vi "Tree_HierarchicalPath_Tests.vi"(11 "error in":errorcluster) -> (15 "error out":errorcluster)   [LabVIEW 2016, in "DronaTest.lvlib"]
uses:
  DronaTest.lvlib
  APIs/Stimulus/ControlValue/SetValueAuto.vi
  APIs/Stimulus/ControlValue/Controls/Tree/SetValueByHierarchicalPath.vi
  APIs/Assert/AssertControlValue/Equal.vi
  APIs/Get/GetControlRef/GetControlRefByPath.vi
  <vilib>/addons/_JKI Toolkits/Caraya/classes/Test/Test.lvclass
  Drona.lvlib
  <vilib>/SLL Toolkit/SLL Debug/SLL Debug.lvlib
  APIs/Assert/AssertControlValue/AssertControlValue.lvlib
  APIs/Stimulus/ControlValue/ControlValue.lvlib
  <vilib>/addons/_JKI Toolkits/Caraya/classes/Assert/Assert.lvclass
  APIs/Stimulus/ControlValue/Controls/Tree/StimulusTree.lvlib
  APIs/Get/GetControlRef/GetControlRef.lvlib
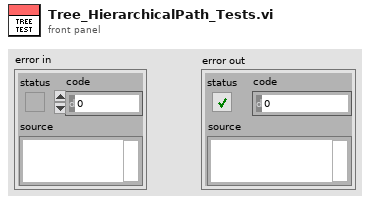
[diagram p1: front panel]
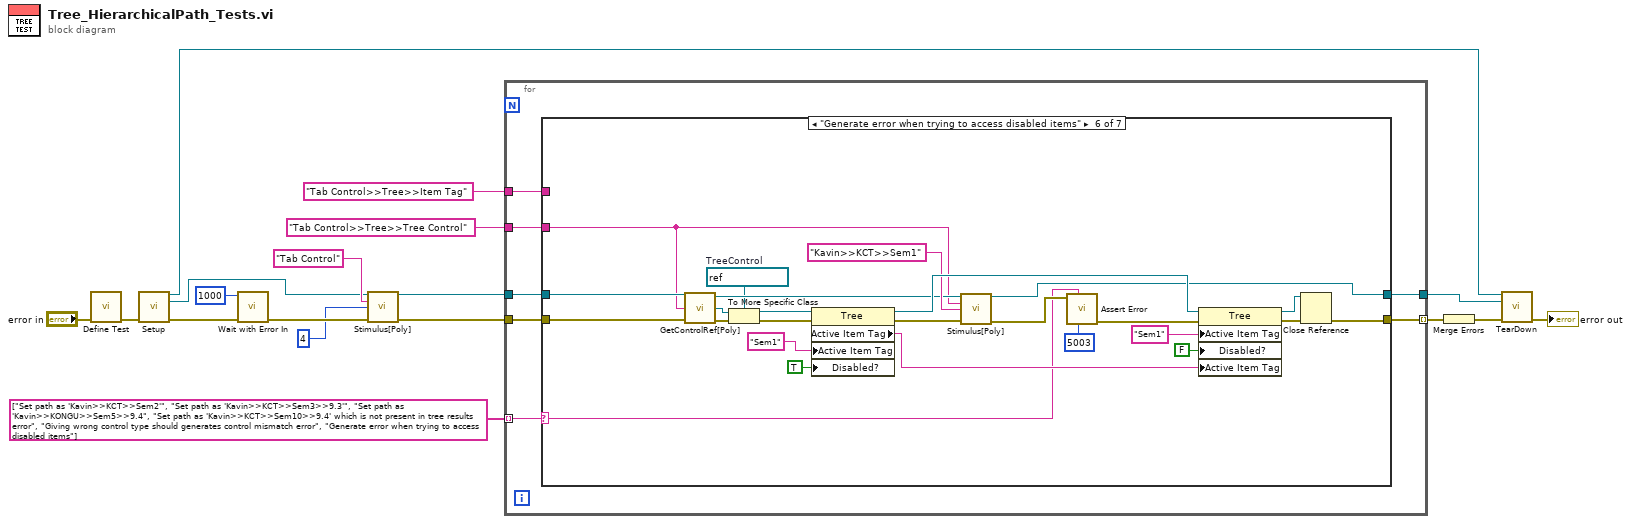
[diagram p0: block diagram]
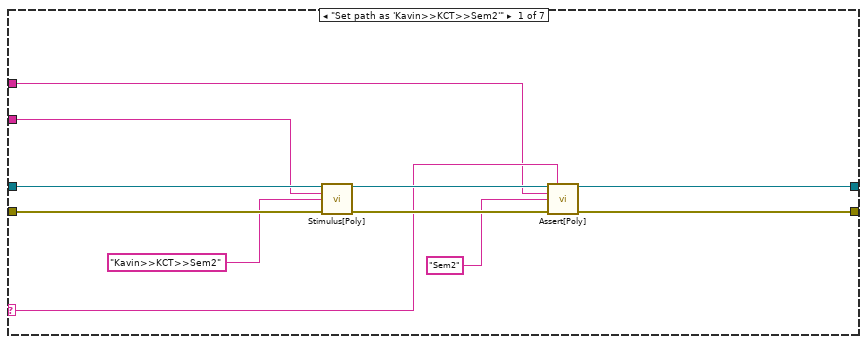
[diagram p2: hidden frame]
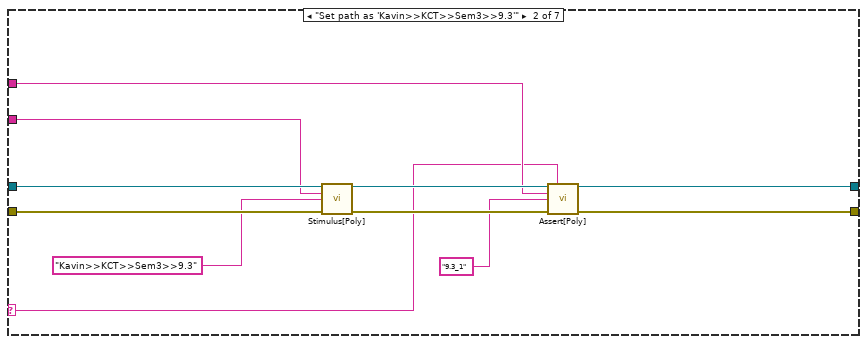
[diagram p3: hidden frame]
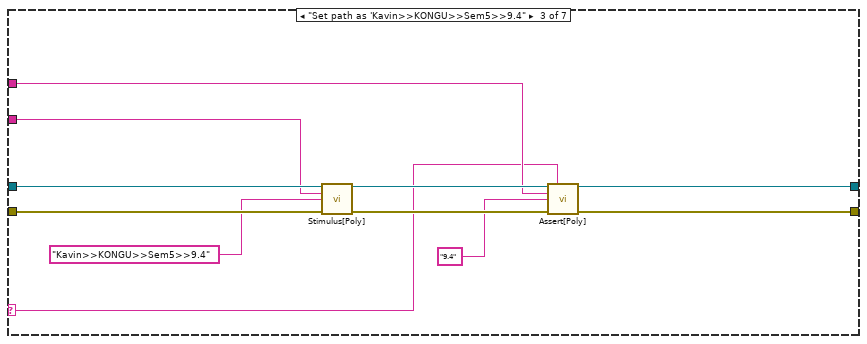
[diagram p4: hidden frame]
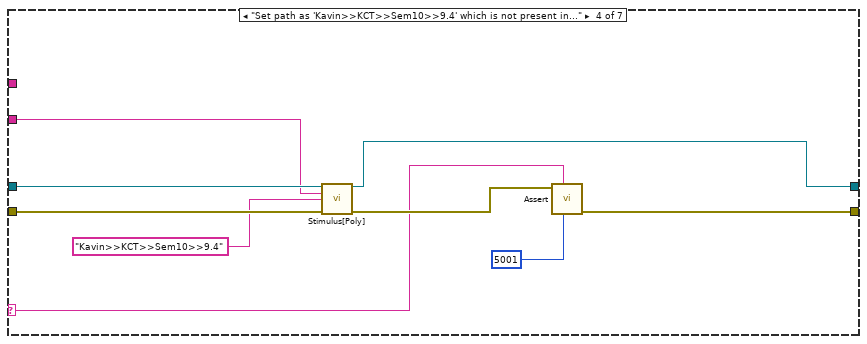
[diagram p5: hidden frame]
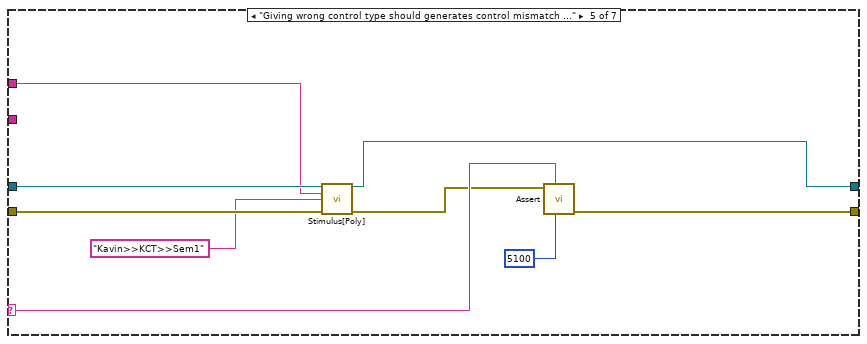
[diagram p6: hidden frame]
diagram:
  n1 = call <vilib>:"Define Test.vi"("error in (no error)"="error in") -> ("error out"=w7:errorcluster)  [unwired: 9 in, 1 out]
  n2 = call "Setup.vi"("error in (no error)"=w7) -> ("Application Ref"=w2:refnum<vi>, "VI out"=w6:refnum<vi>, "error out"=w5:errorcluster)  [unwired: 12 in]
  n3 = call <vilib>:"Wait with Error In.vi"("error in (no error)"=w5, "milliseconds to wait"=u32 1000) -> ("error out"=w16:errorcluster)  [unwired: 9 in]
  n4 = call-poly "Stimulus[Poly].vi"("VI Reference In"=w6, "Control Path"="Tab Control", "Value (Signaling)"=4, "error in"=w16) -> ("VI Reference Out"=w12:refnum<vi>, "error out"=w15:errorcluster)  [unwired: 10 in]
  n5 = for {
    tunnel: w12 -> [w24]
    tunnel: "Tab Control>>Tree>>Tree Control" ("Control Path") -> [w23]
    tunnel: "Tab Control>>Tree>>Item Tag" ("Control Path") -> [w22]
    tunnel: string[] ["Set path as 'Kavin>>KCT>>Sem2'", "Set path as 'Kavin>>KCT>>Sem3>>9.3'", "Set path as 'Kavin>>KONGU>>Sem5>>9.4", "Set path as 'Kavin>>KCT>>Sem10>>9.4' which is not present in tree results error", "Giving wrong control type should generates control mismatch error", "Generate error when trying to access disabled items"] -> [w20] mode=indexing
    tunnel: [w19] -> w3
    tunnel: w15 -> [w25]
    tunnel: [w21] -> w8 mode=indexing
    n6 = case shown="\"Generate error when trying to access disabled items\"" w20 {
      selector: w20 -> [w30 w39 w50 w60 w73 w80 _]
      tunnel: w25 -> [w36 w47 w58 w67 w76 w81 w103]
      tunnel: w24 -> [w35 w46 w57 w66 w75 w82 w102]
      tunnel: w23 -> [w28 w43 w54 w65 _ w79 _]
      tunnel: w22 -> [w29 w42 w53 _ w68 _ _]
      tunnel: [w32 w41 w52 w64 w74 w77 w103] -> w21
      tunnel: [w31 w40 w51 w63 w72 w78 w102] -> w19
      frame "Set path as 'Kavin>>KCT>>Sem2'" {
        n7 = call-poly "Stimulus[Poly].vi"("VI Reference In"=w35, "Control Path"=w28, "Hierarchical Path"="Kavin>>KCT>>Sem2" ("Item Name"), "Error In"=w36) -> ("VI Reference Out"=w33:refnum<vi>, "Error Out"=w34:errorcluster)  [unwired: 10 in]
        n8 = call-poly "Assert[Poly].vi"("VI Reference In"=w33, "Test Label"=w30, "Control Path"=w29, "Control Value"="Sem2", "Error In"=w34) -> ("VI Reference Out"=w31:refnum<vi>, "Error Out"=w32:errorcluster)  [unwired: 8 in, 1 out]
      }
      frame "Set path as 'Kavin>>KCT>>Sem3>>9.3'" {
        n9 = call-poly "Stimulus[Poly].vi"("VI Reference In"=w46, "Control Path"=w43, "Hierarchical Path"="Kavin>>KCT>>Sem3>>9.3" ("Item Name"), "Error In"=w47) -> ("VI Reference Out"=w44:refnum<vi>, "Error Out"=w45:errorcluster)  [unwired: 10 in]
        n10 = call-poly "Assert[Poly].vi"("VI Reference In"=w44, "Test Label"=w39, "Control Path"=w42, "Control Value"="9.3_1", "Error In"=w45) -> ("VI Reference Out"=w40:refnum<vi>, "Error Out"=w41:errorcluster)  [unwired: 8 in, 1 out]
      }
      frame "Set path as 'Kavin>>KONGU>>Sem5>>9.4" {
        n11 = call-poly "Stimulus[Poly].vi"("VI Reference In"=w57, "Control Path"=w54, "Hierarchical Path"="Kavin>>KONGU>>Sem5>>9.4" ("Item Name"), "Error In"=w58) -> ("VI Reference Out"=w55:refnum<vi>, "Error Out"=w56:errorcluster)  [unwired: 10 in]
        n12 = call-poly "Assert[Poly].vi"("VI Reference In"=w55, "Test Label"=w50, "Control Path"=w53, "Control Value"="9.4" ("Item Name"), "Error In"=w56) -> ("VI Reference Out"=w51:refnum<vi>, "Error Out"=w52:errorcluster)  [unwired: 8 in, 1 out]
      }
      frame "Set path as 'Kavin>>KCT>>Sem10>>9.4' which is not present in tree results error" {
        n13 = call-poly "Stimulus[Poly].vi"("VI Reference In"=w66, "Control Path"=w65, "Hierarchical Path"="Kavin>>KCT>>Sem10>>9.4" ("Item Name"), "Error In"=w67) -> ("VI Reference Out"=w63:refnum<vi>, "Error Out"=w61:errorcluster)  [unwired: 10 in]
        n14 = call-poly <vilib>:"Assert.vi"("error code (1)"=5001, "Label"=w60, "Error?"=w61) -> ("error out"=w64:errorcluster)  [unwired: 7 in, 1 out]
      }
      frame "Giving wrong control type should generates control mismatch error" {
        n15 = call-poly "Stimulus[Poly].vi"("VI Reference In"=w75, "Control Path"=w68, "Hierarchical Path"="Kavin>>KCT>>Sem1" ("Item Name"), "Error In"=w76) -> ("VI Reference Out"=w72:refnum<vi>, "Error Out"=w70:errorcluster)  [unwired: 10 in]
        n16 = call-poly <vilib>:"Assert.vi"("error code (1)"=5100, "Label"=w73, "Error?"=w70) -> ("error out"=w74:errorcluster)  [unwired: 7 in, 1 out]
      }
      frame "Generate error when trying to access disabled items" {
        w86 = refnum<vi> refnum  # TreeControl
        n17 = call-poly "GetControlRef[Poly].vi"("VI Reference In"=w82, "Control Path"=w79, "error In"=w81) -> ("VI Reference Out"=w93:refnum<vi>, "Ctl Refnum"=w85:refnum<vi>, "error out"=w83:errorcluster)  [unwired: 10 in]
        n18 = To More Specific Class(target class=w86, reference=w85, error in=w83) -> (specific class reference=w87:refnum<vi>, error out=w84:errorcluster)
        n19 = property class="Tree"(reference=w87, error in=w84, "Active Item Tag"="Sem1" ("Active Item:Tag"), "Disabled?"=TRUE ("Active Item:Disabled?")) -> (reference out=w98:refnum<vi>, error out=w92:errorcluster, "Active Item Tag"=w99:string)
        n20 = call-poly "Stimulus[Poly].vi"("VI Reference In"=w93, "Control Path"=w79, "Hierarchical Path"="Kavin>>KCT>>Sem1" ("Item Tag"), "Error In"=w92) -> ("VI Reference Out"=w78:refnum<vi>, "Error Out"=w95:errorcluster)  [unwired: 10 in]
        n21 = call <vilib>:"Assert Error.vi"("error code (1)"=5003, "Label"=w80, "Error?"=w95) -> ("error out"=w96:errorcluster)  [unwired: 7 in, 1 out]
        n22 = property class="Tree"(reference=w98, error in=w96, "Active Item Tag"="Sem1" ("Active Item:Tag"), "Disabled?"=FALSE ("Active Item:Disabled?"), "Active Item Tag"=w99) -> (reference out=w91:refnum<vi>, error out=w90:errorcluster)
        n23 = Close Reference(reference=w91, error in (no error)=w90) -> (error out=w77:errorcluster)
      }
      frame Default {
      }
    }
  }
  n24 = Merge Errors(w8) -> (w4:errorcluster)
  n25 = call "TearDown.vi"("Application Ref"=w2, "VI in"=w3, "error in (no error)"=w4) -> ("error out"=→"error out":errorcluster)  [unwired: 12 in]
